vi "Save_interim_img_tiff.vi"() -> ()   [LabVIEW 2020]
uses:
  <vilib>/vision/NI_Vision_Development_Module.lvlib
panel:
  out "Elapsed time [ms]":u32
  in  "h":i32=10 min=1 max=5000 step=1
  in  "w":i32=1 min=1 max=5000 step=1
  out "error out":errorcluster
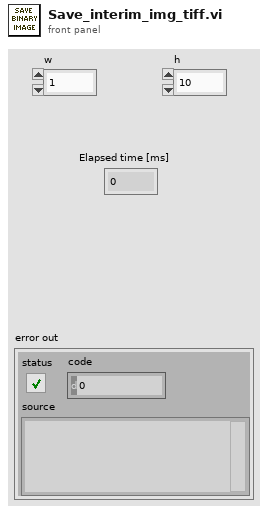
[diagram p1: front panel]
types:
  T1 = cluster{"Rows Per Strip":i32, "Photometric":i32, "Compression Type":i32}
  T2 = typedef "Image Type" = u32
  T3 = typedef "IMAQ Image.ctl" = refnum<image>
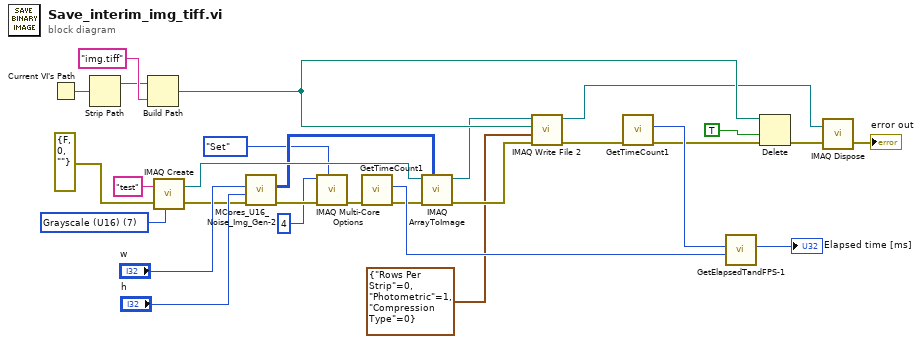
[diagram p0: block diagram]
diagram:
  w17 = T2 7 items=["Grayscale (U8)", "Grayscale (I16)", "Grayscale (SGL)", "Complex (CSG)", "RGB (U32)", "HSL (U32)", "RGB (U64)", "Grayscale (U16)"] ("Image Type")
  n1 = Current VI's Path() -> (path=w29:path)
  n2 = Strip Path(path=w29) -> (stripped path=w27:path)  [unwired: 1 out]
  n3 = Build Path(base path=w27, name or relative path="img.tiff" ("string")) -> (appended path=w13:path)
  n4 = call "IMAQ Create"("Image Name"="test", "Image Type"=w17, "error in (no error)"=errorcluster {"status"=FALSE, "code"=0, "source"=""}) -> ("New Image"=w10:T3, "error out"=w18:errorcluster)  [unwired: 2 in]
  n5 = call "MCores_U16_Noise_Img_Gen-2.vi"("error IN"=w18, "[IN] Width"="h", "[IN] Height"="w") -> ("error OUT"=w5:errorcluster, "[OUT] U16 Pixel Img"=w9:u16[][])  [unwired: 7 in]
  n6 = call "IMAQ Multi-Core Options"("Get/Set Number of Cores (Get)"=enum32{"Get", "Set", "Set Max Available"}."Set", "error in (no error)"=w5, "Specified Number of Cores"=u32 4) -> ("error out"=w4:errorcluster)  [unwired: 7 in, 1 out]
  n7 = call "GetTimeCount1.vi"("error IN"=w4) -> ("error OUT"=w12:errorcluster, "[OUT] Timer Count"=w23:u32)  [unwired: 9 in]
  n8 = call "IMAQ ArrayToImage"("Image Pixels (U16)"=w9, "error in (no error)"=w12, "Image"=w10) -> ("error out"=w11:errorcluster, "Image Out"=w8:T3)  [unwired: 7 in]
  n9 = call-poly "IMAQ Write File 2"("error in (no error)"=w11, "TIFF Options"=T1 {"Rows Per Strip"=0, "Photometric"=1, "Compression Type"=0}, "File Path"=w13, "Image"=w8) -> ("error out"=w7:errorcluster, "Image Out (duplicate)"=w6:T3)  [unwired: 6 in]
  n10 = call "GetTimeCount1.vi"("error IN"=w7) -> ("error OUT"=w21:errorcluster, "[OUT] Timer Count"=w24:u32)  [unwired: 9 in]
  n11 = call "GetElapsedTandFPS-1.vi"("[IN] Timer Count Before ALL [ms]"=w23, "[IN] Timer Count After ALL [ms]"=w24) -> ("[OUT] Elapsed time [ms]"=→"Elapsed time [ms]":u32)  [unwired: 3 in, 2 out]
  n12 = Delete(path (use dialog)=w13, confirm (F)=TRUE, error in=w21) -> (error out=w15:errorcluster)  [unwired: 2 in, 2 out]
  n13 = call "IMAQ Dispose"("Image"=w6, "error in (no error)"=w15) -> ("error out"=→"error out":errorcluster)  [unwired: 4 in]
